vi "4pinSensor.vi"(8 "Echo":refnum<k21>="ConnectorA/DIO9", 9 "Trigger":refnum<k21>="ConnectorA/DIO8", 10 "Count(Ticks)":u32=20, 11 "Count(Ticks) 2":u32=50) -> (3 "Time":u32)   [LabVIEW 2014]
uses:
  <vilib>/rvi/eio/common/nirviEmuTemplateMethod_errors.vi
  <vilib>/rvi/Emulation/niFpgaGetClockAttributes.vi
  <vilib>/rvi/Emulation/niFpgaSctlEmulationGetInTimedLoop.vi
  <vilib>/rvi/Emulation/niFpgaEmulationReportErrorSimple.vi
  <vilib>/rvi/Emulation/niFpgaCriticalErrorInLSC.vi
  <vilib>/eio/EIONode/EIONode.xnode
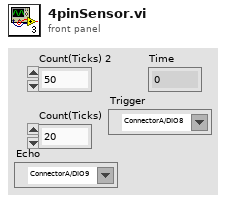
[diagram p1: front panel]
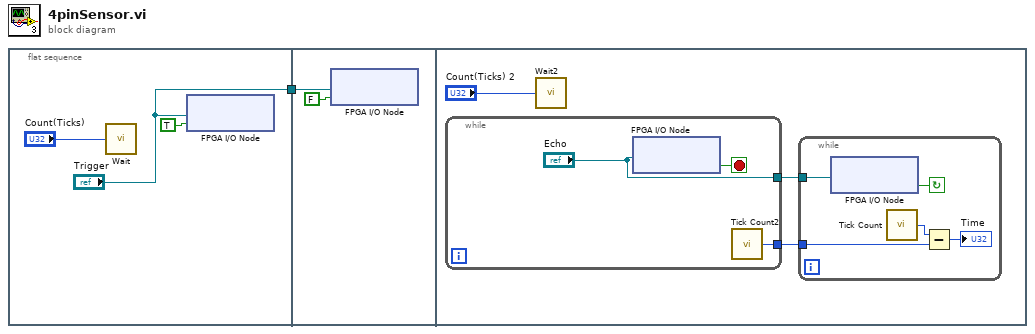
[diagram p0: block diagram]
diagram:
  n1 = flat-sequence {
    tunnel: ["Trigger"] -> w1
    tunnel: w1 -> [w5]
    frame #0 {
      n2 = call "Wait"("Count(uSec)"="Count(Ticks)") -> ()  [unwired: 1 out]
      n3 = xnode "FPGA I/O Node"("I/O Item"=TRUE, "FPGA I/O In"="Trigger") -> ()  [unwired: 1 out]
    }
    frame #1 {
      n4 = xnode "FPGA I/O Node"("I/O Item"=FALSE, "FPGA I/O In"=w5) -> ()  [unwired: 1 out]
    }
    frame #2 {
      n5 = while {
        tunnel: ["Echo"] -> w8
        tunnel: [w10] -> w7
        stop <- w12 stop-if-true
        n6 = xnode "FPGA I/O Node"("FPGA I/O In"="Echo") -> ("I/O Item"=w12:bool)  [unwired: 1 out]
        n7 = call "Tick Count2"() -> ("Tick Count(uSec)"=w10:u32)
      }
      n8 = call "Wait2"("Count(mSec)"="Count(Ticks) 2") -> ()  [unwired: 1 out]
      n9 = while {
        tunnel: w8 -> [w16]
        tunnel: w7 -> [w14]
        stop <- w17 continue-if-true
        n10 = xnode "FPGA I/O Node"("FPGA I/O In"=w16) -> ("I/O Item"=w17:bool)  [unwired: 1 out]
        n11 = call "Tick Count"() -> ("Tick Count(uSec)"=w15:u32)
        n12 = Subtract(x=w15, y=w14) -> (x-y=→"Time":u32)
      }
    }
  }
